vi "images.vi"(0 "Camera in":refnum<class "Camera.lvclass">, 1 "start_index":u32, 5 "data_format":T3(ring)=enum."Mono16", 7 "image_count":u32, 9 "crop":cluster{"x0":u64, "y0":u64, "x1":u64, "y1":u64}={"x0"=1, "y0"=1, "x1"=18446744073709551615, "y1"=18446744073709551615}, 11 "error in (no error)":errorcluster, 12 "PCO_Recorder_CompressionParams":T5={"dGainK"=nan, "dDarkNoise_e"=nan, "dDSNU_e"=nan, "dPRNU_pct"=nan, "dLightSourceNoise_pct"=0.0}) -> (2 "timestamp_list":T4(array[cluster]) {"lvTimestamp" format="%<%.6X\n%x>T"}, 3 "meta_data_list":T1(array[cluster]), 4 "Camera out":refnum<class "Camera.lvclass">, 6 "image_list (U8)":u8[][][](array[numeric]), 8 "image_list (U32)":u32[][][](array[numeric]), 10 "image_list (U64)":T2(array[cluster]), 13 "raw_image_8_list (U8)":u8[][][](array[numeric]), 14 "raw_image_list (U16)":u16[][][](array[numeric]), 15 "error out":errorcluster)   [LabVIEW 2019, in "Camera.lvclass"]
doc: "Get a series of images from the recorder as a 3D array. The positions of the images to query are defined by start_index and image_count. \nThis array is shaped depending on the\nresolution and ROI of the image and the number of recorded images. The data is stored in the\norder of image, row, column. The data format determines which output is valid, but the raw_image(16) output is always valid."
uses:
  Camera.lvclass
  Camera.lvclass/Camera.ctl
  pco.recorder/Recorder.lvlib
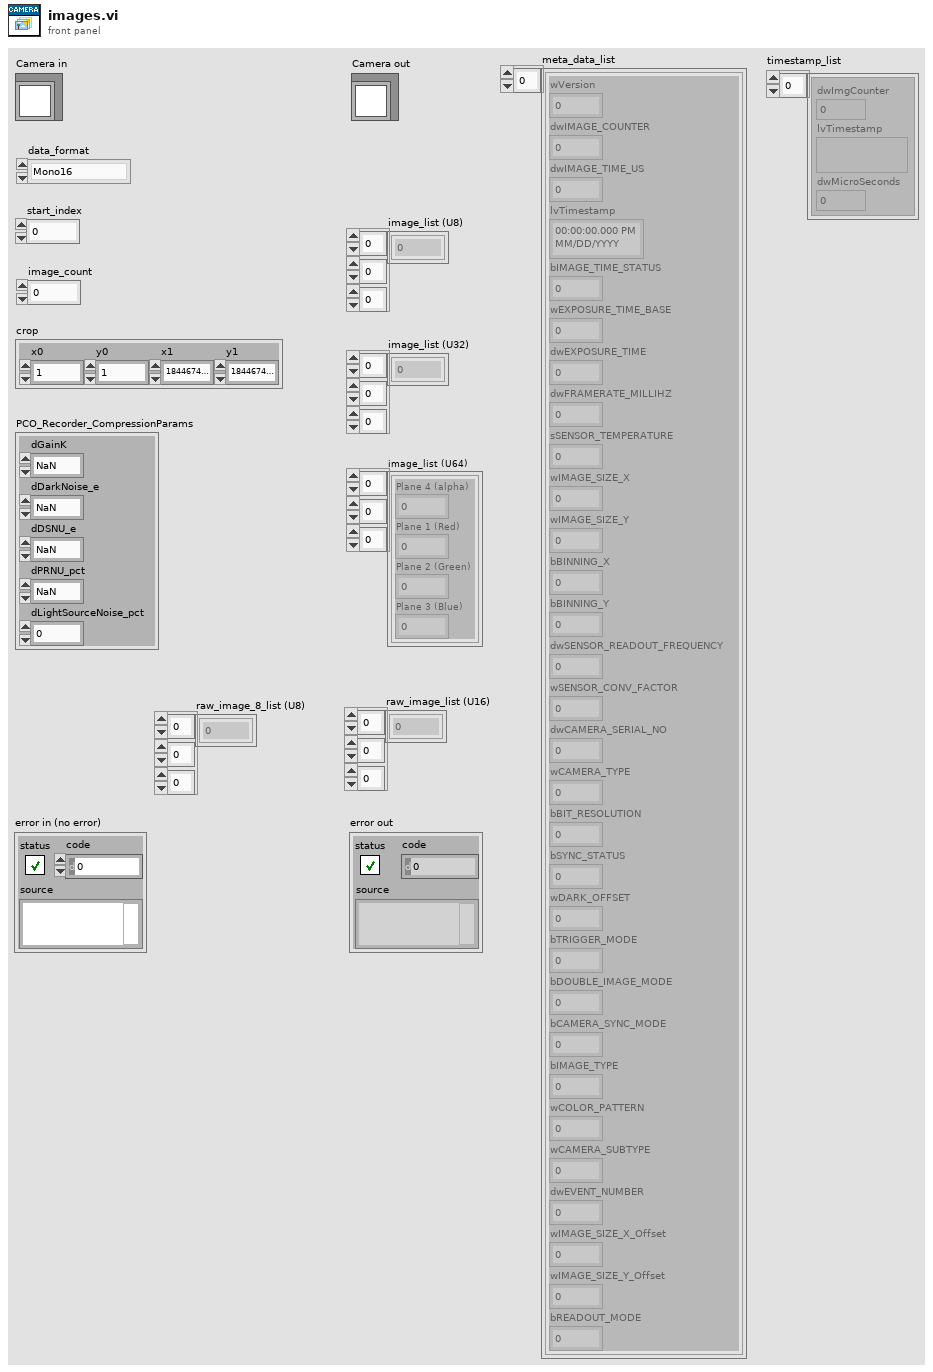
[diagram p1: front panel]
types:
  T1 = cluster{"wVersion":u16, "dwIMAGE_COUNTER":u32, "dwIMAGE_TIME_US":u32, "lvTimestamp":timestamp, "bIMAGE_TIME_STATUS":u8, "wEXPOSURE_TIME_BASE":u16, "dwEXPOSURE_TIME":u32, "dwFRAMERATE_MILLIHZ":u32, "sSENSOR_TEMPERATURE":i16, "wIMAGE_SIZE_X":u16, "wIMAGE_SIZE_Y":u16, "bBINNING_X":u8, "bBINNING_Y":u8, "dwSENSOR_READOUT_FREQUENCY":u32, "wSENSOR_CONV_FACTOR":u16, "dwCAMERA_SERIAL_NO":u32, "wCAMERA_TYPE":u16, "bBIT_RESOLUTION":u8, "bSYNC_STATUS":u8, "wDARK_OFFSET":u16, "bTRIGGER_MODE":u8, "bDOUBLE_IMAGE_MODE":u8, "bCAMERA_SYNC_MODE":u8, "bIMAGE_TYPE":u8, "wCOLOR_PATTERN":u16, "wCAMERA_SUBTYPE":u16, "dwEVENT_NUMBER":u32, "wIMAGE_SIZE_X_Offset":u16, "wIMAGE_SIZE_Y_Offset":u16, "bREADOUT_MODE":u8}[]
  T2 = cluster{"Plane 4 (alpha)":u16, "Plane 1 (Red)":u16, "Plane 2 (Green)":u16, "Plane 3 (Blue)":u16}[][][]
  T3 = enum16{"Undefined", "Mono8", "Mono16", "BGRA8", "RGBA8", "BGRA16", "RGBA16", "CompressedMono8"}
  T4 = cluster{"dwImgCounter":u32, "lvTimestamp":timestamp, "dwMicroSeconds":u32}[]
  T5 = cluster{"dGainK":dbl, "dDarkNoise_e":dbl, "dDSNU_e":dbl, "dPRNU_pct":dbl, "dLightSourceNoise_pct":dbl}
  T6 = cluster{"dwImgCounter":u32, "lvTimestamp":timestamp, "dwMicroSeconds":u32}
  T7 = cluster{"wVersion":u16, "dwIMAGE_COUNTER":u32, "dwIMAGE_TIME_US":u32, "lvTimestamp":timestamp, "bIMAGE_TIME_STATUS":u8, "wEXPOSURE_TIME_BASE":u16, "dwEXPOSURE_TIME":u32, "dwFRAMERATE_MILLIHZ":u32, "sSENSOR_TEMPERATURE":i16, "wIMAGE_SIZE_X":u16, "wIMAGE_SIZE_Y":u16, "bBINNING_X":u8, "bBINNING_Y":u8, "dwSENSOR_READOUT_FREQUENCY":u32, "wSENSOR_CONV_FACTOR":u16, "dwCAMERA_SERIAL_NO":u32, "wCAMERA_TYPE":u16, "bBIT_RESOLUTION":u8, "bSYNC_STATUS":u8, "wDARK_OFFSET":u16, "bTRIGGER_MODE":u8, "bDOUBLE_IMAGE_MODE":u8, "bCAMERA_SYNC_MODE":u8, "bIMAGE_TYPE":u8, "wCOLOR_PATTERN":u16, "wCAMERA_SUBTYPE":u16, "dwEVENT_NUMBER":u32, "wIMAGE_SIZE_X_Offset":u16, "wIMAGE_SIZE_Y_Offset":u16, "bREADOUT_MODE":u8}
  T8 = cluster{"Plane 4 (alpha)":u16, "Plane 1 (Red)":u16, "Plane 2 (Green)":u16, "Plane 3 (Blue)":u16}[][]
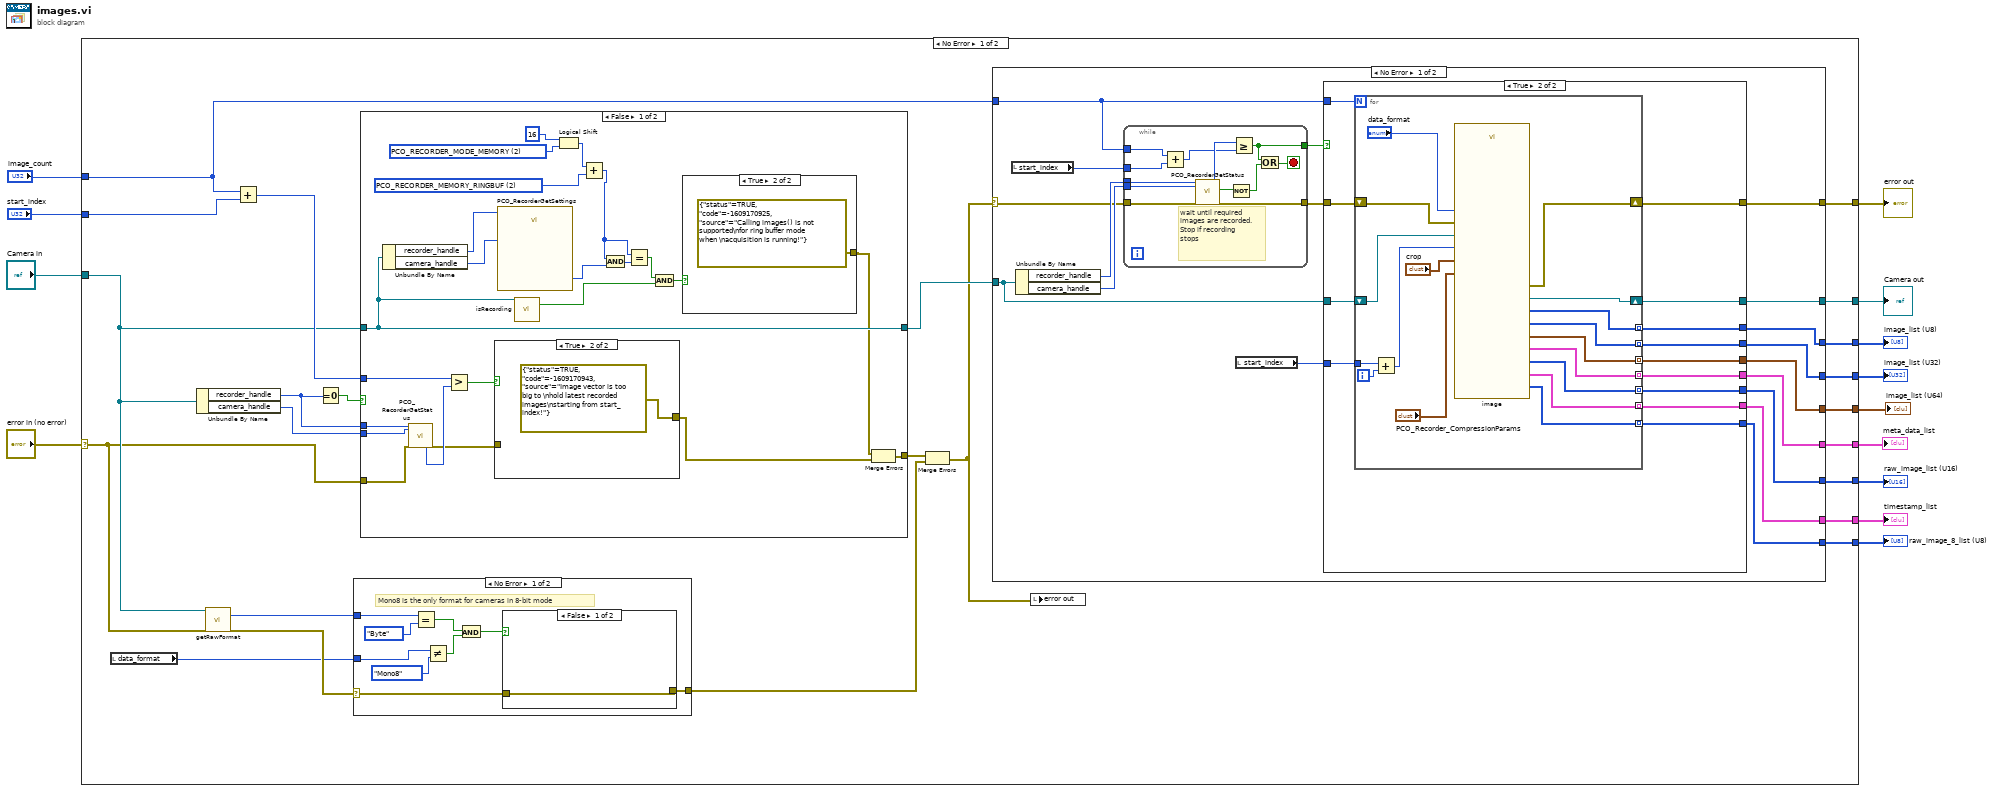
[diagram p0: block diagram]
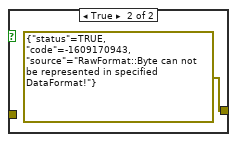
[diagram p2: hidden frame]
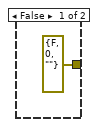
[diagram p4: hidden frame]
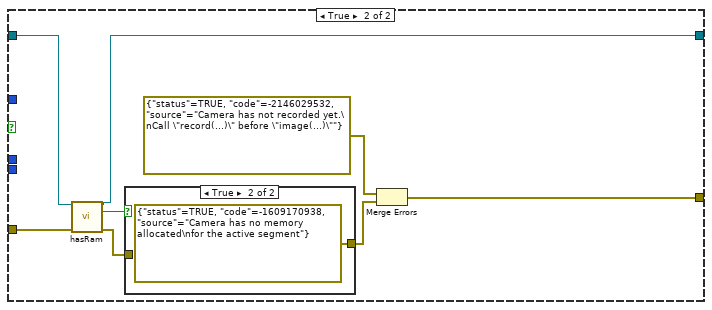
[diagram p6: hidden frame]
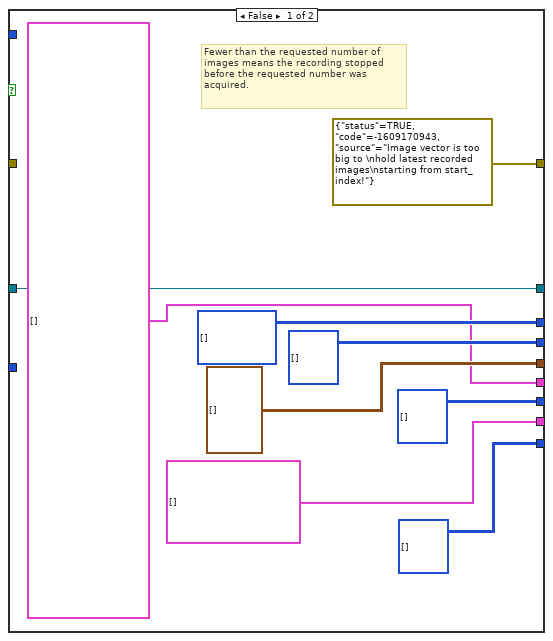
[diagram p8: hidden frame]
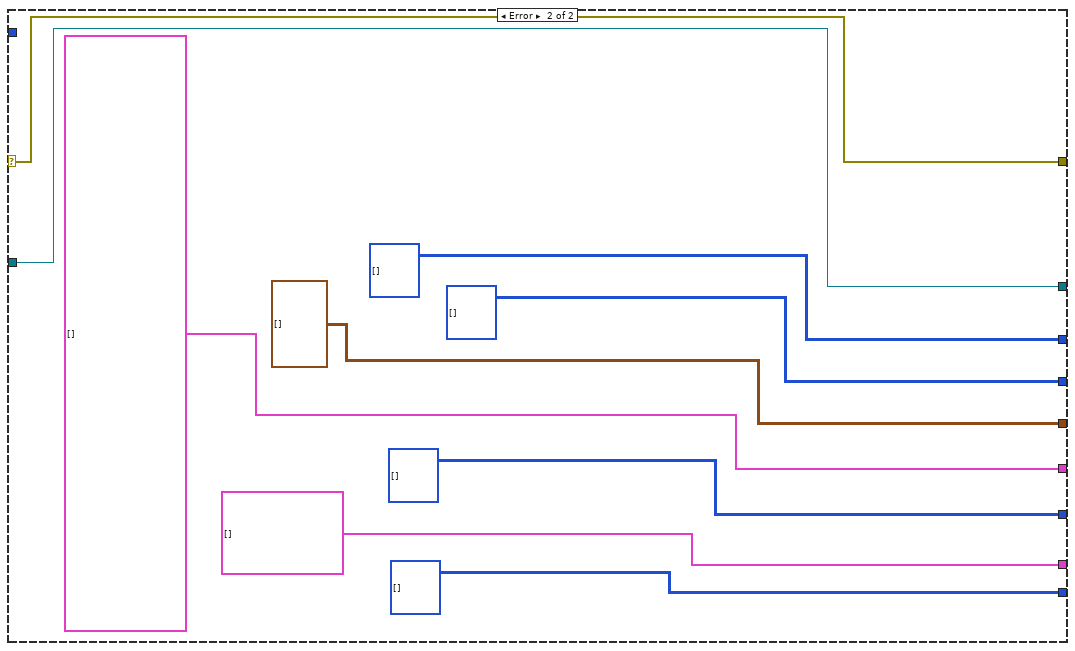
[diagram p9: hidden frame]
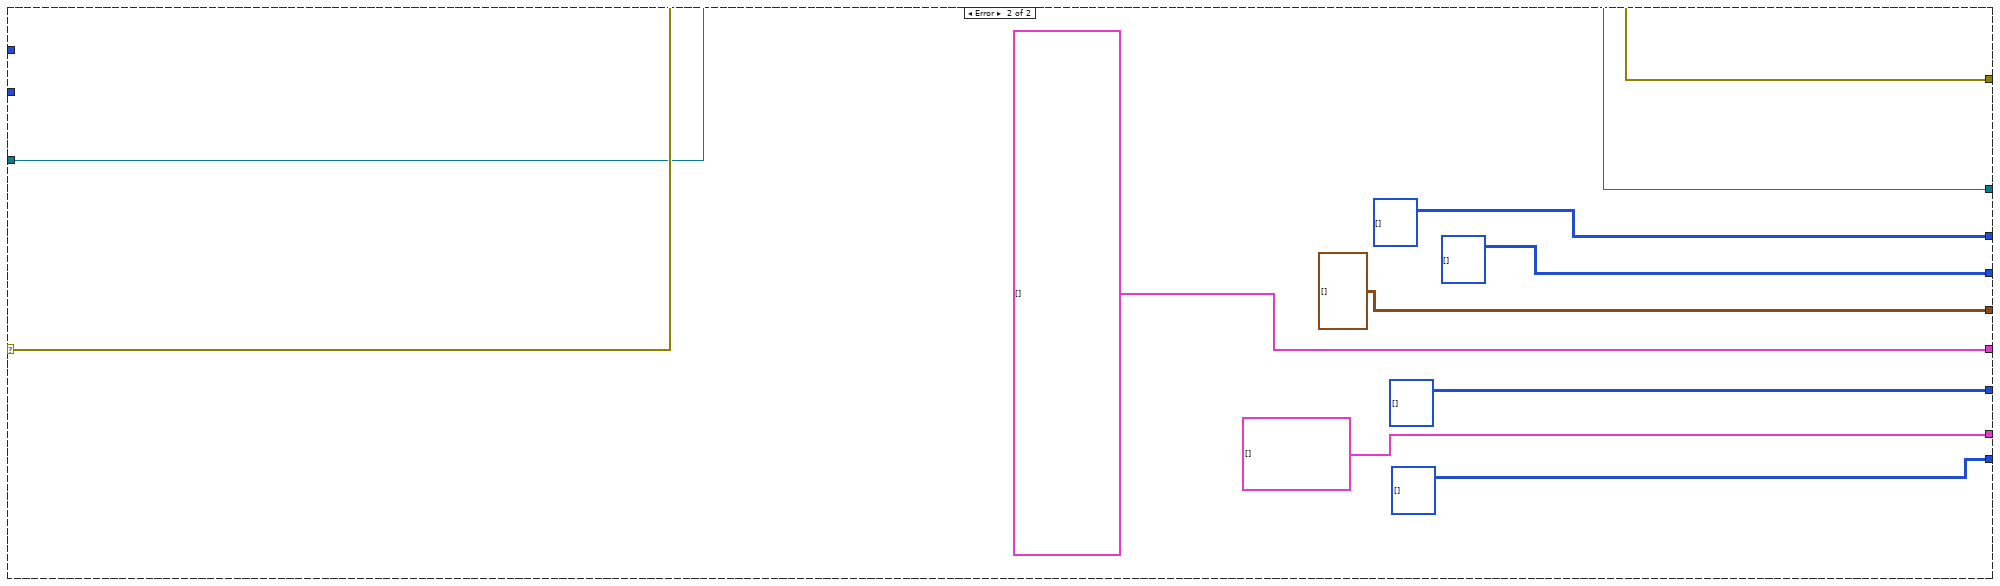
[diagram p10: hidden frame]
diagram:
  n1 = case shown="No Error" "error in (no error)" {
    selector: "error in (no error)" -> [w15 w171]
    tunnel: "Camera in" -> [w16 w170]
    tunnel: "image_count" -> [w29 _]
    tunnel: [w37 w171] -> w10
    tunnel: [w36 w170] -> w9
    tunnel: [w35 u8[][][] [] ("image (U8)")] -> w8
    tunnel: [w34 u32[][][] [] ("image (U16)")] -> w7
    tunnel: [w33 T1 [] ("meta_data_list")] -> w1
    tunnel: [w32 u16[][][] [] ("raw_image (U16)")] -> w6
    tunnel: [w31 T4 []] -> w5
    tunnel: "start_index" -> [w30 _]
    tunnel: [w28 T2 [] ("image (U64)")] -> w3
    tunnel: [w14 u8[][][] [] ("raw_image (U16)")] -> w2
    frame No Error {
      n2 = local read "data_format"() -> (w19:T3)
      n3 = Unbundle By Name(w16) -> ("recorder_handle"=w26:u64, "camera_handle"=w25:u64)
      n4 = call-dynamic "getRawFormat.vi"("Camera in"=w16, "error in (no error)"=w15) -> ("rawFormat"=w20:enum16{"Word", "Byte"}, "error out"=w21:errorcluster)  [unwired: 11 in, 1 out]
      n5 = Add(x=w29, y=w30) -> (x+y=w24:u32)
      n6 = Equal To 0?(x=w26) -> (x = 0?=w27:bool)
      n7 = case shown="No Error" w21 {
        selector: w21 -> [w39 w49]
        tunnel: w20 -> [w46 _]
        tunnel: w19 -> [w44 _]
        tunnel: [w38 w49] -> w17
        frame No Error {
          # "Mono8 is the only format for cameras in 8-bit mode"
          n8 = Equal?(x=w46, y=enum16{"Word", "Byte"}."Byte" ("rawFormat")) -> (x = y?=w42:bool)
          n9 = Not Equal?(x=w44, y=T3."Mono8" ("data_format")) -> (x != y?=w41:bool)
          n10 = And(x=w42, y=w41) -> (x .and. y?=w40:bool)
          n11 = case shown="False" w40 {
            tunnel: w39 -> [w47 _]
            tunnel: [w47 errorcluster {"status"=TRUE, "code"=-1609170943, "source"="RawFormat::Byte can not be represented in specified DataFormat!"} ("error constant")] -> w38
            frame False {
            }
            frame True {
            }
          }
        }
        frame Error {
        }
      }
      n12 = case shown="False" w27 {
        tunnel: w15 -> [w72 w80]
        tunnel: w16 -> [w59 w79]
        tunnel: [w57 w78] -> w22
        tunnel: w26 -> [w71 _]
        tunnel: w25 -> [w70 _]
        tunnel: w24 -> [w69 _]
        tunnel: [w59 w77] -> w23
        frame False {
          w50 = u32 2 items=["PCO_RECORDER_MODE_FILE"=1, "PCO_RECORDER_MODE_MEMORY"=2, "PCO_RECORDER_MODE_CAMRAM"=3] ("wRecMode")
          w62 = u32 2 items=["PCO_RECORDER_MEMORY_SEQUENCE"=1, "PCO_RECORDER_MEMORY_RINGBUF"=2, "PCO_RECORDER_MEMORY_FIFO"=3] ("wRecType")
          n13 = Unbundle By Name(w59) -> ("recorder_handle"=w65:u64, "camera_handle"=w64:u64)
          n14 = call "PCO_RecorderGetStatus.vi"("phRec"=w71, "phCam"=w70, "error in (no error)"=w72) -> ("dwReqImgCount"=w68:u32, "error out"=w66:errorcluster)  [unwired: 5 in, 10 out]
          n15 = Greater?(x=w69, y=w68) -> (0:w67:bool)
          n16 = case shown="True" w67 {
            tunnel: [w75 errorcluster {"status"=TRUE, "code"=-1609170943, "source"="Image vector is too big to \nhold latest recorded images\nstarting from start_index!"} ("error constant")] -> w56
            tunnel: w66 -> [w75 _]
            frame False {
            }
            frame True {
            }
          }
          n17 = call "PCO_RecorderGetSettings.vi"("phRec"=w65, "phCam"=w64) -> ("dwRecMode"=w54:u32)  [unwired: 5 in, 8 out]
          n18 = call-dynamic "isRecording.vi"("Camera in"=w59) -> ("recording"=w60:bool)  [unwired: 12 in, 2 out]
          n19 = Logical Shift(y=u32 16 ("x"), x=w50) -> (x << y=w63:u32)
          n20 = Add(x=w63, y=w62) -> (x+y=w52:u32)
          n21 = And(x=w52, y=w54) -> (x .and. y?=w53:u32)
          n22 = Equal?(x=w52, y=w53) -> (x = y?=w61:bool)
          n23 = And(x=w61, y=w60) -> (x .and. y?=w58:bool)
          n24 = case shown="True" w58 {
            tunnel: [errorcluster {"status"=FALSE, "code"=0, "source"=""} ("error constant") errorcluster {"status"=TRUE, "code"=-1609170925, "source"="Calling images() is not supported\nfor ring buffer mode when \nacquisition is running!"} ("error constant")] -> w55
            frame False {
            }
            frame True {
            }
          }
          n25 = Merge Errors(w55, w56) -> (w57:errorcluster)
        }
        frame True {
          n26 = call-dynamic "hasRam.vi"("Camera in"=w79, "error in (no error)"=w80) -> ("Camera out"=w77:refnum<class "Camera.lvclass">, "hasRam"=w84:bool, "error out"=w83:errorcluster)  [unwired: 11 in]
          n27 = case shown="True" w84 {
            tunnel: w83 -> [w85 _]
            tunnel: [w85 errorcluster {"status"=TRUE, "code"=-1609170938, "source"="Camera has no memory allocated\nfor the active segment"} ("error constant")] -> w81
            frame False {
            }
            frame True {
            }
          }
          n28 = Merge Errors(errorcluster {"status"=TRUE, "code"=-2146029532, "source"="Camera has not recorded yet.\nCall \"record(...)\" before \"image(...)\""} ("error constant"), w81) -> (w78:errorcluster)
        }
      }
      n29 = Merge Errors(w22, w17) -> (w18:errorcluster)
      n30 = case shown="No Error" w18 {
        selector: w18 -> [w92 w164]
        tunnel: w29 -> [w102 _]
        tunnel: w23 -> [w101 w163]
        tunnel: [w99 w164] -> w37
        tunnel: [w98 w163] -> w36
        tunnel: [w93 u8[][][] [] ("image (U8)")] -> w35
        tunnel: [w97 u32[][][] [] ("image (U16)")] -> w34
        tunnel: [w89 T2 [] ("image (U64)")] -> w28
        tunnel: [w96 T1 [] ("meta_data_list")] -> w33
        tunnel: [w95 u16[][][] [] ("raw_image (U16)")] -> w32
        tunnel: [w94 T4 []] -> w31
        tunnel: [w87 u8[][][] [] ("raw_image (U16)")] -> w14
        frame No Error {
          n31 = local read "start_index"() -> (w91:u32)
          n32 = Unbundle By Name(w101) -> ("recorder_handle"=w104:u64, "camera_handle"=w103:u64)
          n33 = while {
            tunnel: w104 -> [w155]
            tunnel: w103 -> [w154]
            tunnel: w92 -> [w153]
            tunnel: w102 -> [w150]
            tunnel: [w152] -> w100
            tunnel: w91 -> [w149]
            tunnel: [w144] -> w88
            stop <- w145 stop-if-true
            # "wait until required \nimages are recorded. Stop if recording stops"
            n34 = Add(x=w150, y=w149) -> (x+y=w148:u32)
            n35 = call "PCO_RecorderGetStatus.vi"("phRec"=w155, "phCam"=w154, "error in (no error)"=w153) -> ("dwProcImgCount"=w151:u32, "bIsRunning"=w147:bool, "error out"=w152:errorcluster)  [unwired: 5 in, 9 out]
            n36 = Not(x=w147) -> (.not. x?=w146:bool)
            n37 = Greater Or Equal?(x=w151, y=w148) -> (x >= y?=w144:bool)
            n38 = Or(x=w144, y=w146) -> (x .or. y?=w145:bool)
          }
          n39 = local read "start_index"() -> (w90:u32)
          n40 = case shown="True" w88 {
            tunnel: w102 -> [_ w126]
            tunnel: w101 -> [w112 w125]
            tunnel: w100 -> [_ w124]
            tunnel: [errorcluster {"status"=TRUE, "code"=-1609170943, "source"="Image vector is too big to \nhold latest recorded images\nstarting from start_index!"} ("error constant") w123] -> w99
            tunnel: [w112 w122] -> w98
            tunnel: [u32[][][] [] ("image (U32)") w121] -> w97
            tunnel: [T1 [] ("meta_data_list") w120] -> w96
            tunnel: [u16[][][] [] ("raw_image (U16)") w119] -> w95
            tunnel: [T4 [] w118] -> w94
            tunnel: [u8[][][] [] ("image (U8)") w117] -> w93
            tunnel: w90 -> [_ w116]
            tunnel: [T2 [] ("image (U64)") w115] -> w89
            tunnel: [u8[][][] [] ("raw_image (U16)") w114] -> w87
            frame False {
              # "Fewer than the requested number of images means the recording stopped before the requested number was acquired."
            }
            frame True {
              n41 = for {
                N: w126 -> [_]
                shift-right: [w140] -> w123
                shift-left: w124 -> [w141]
                shift-right: [w139] -> w122
                shift-left: w125 -> [w143]
                tunnel: [w138] -> w121 mode=indexing
                tunnel: [w137] -> w117 mode=indexing
                tunnel: [w136] -> w115 mode=indexing
                tunnel: [w135] -> w120 mode=indexing
                tunnel: [w134] -> w119 mode=indexing
                tunnel: [w131] -> w118 mode=indexing
                tunnel: w116 -> [w129]
                tunnel: [w127] -> w114 mode=indexing
                i -> [w130]
                n42 = Add(x=w129, y=w130) -> (x+y=w128:u32)
                n43 = call-dynamic "image.vi"("Camera in"=w143, "data_format"="data_format", "image_index"=w128, "crop"="crop", "error in (no error)"=w141, "PCO_Recorder_CompressionParams"="PCO_Recorder_CompressionParams") -> ("timestamp"=w131:T6, "meta_data"=w135:T7, "Camera out"=w139:refnum<class "Camera.lvclass">, "image (U8)"=w137:u8[][], "image (U32)"=w138:u32[][], "image (U64)"=w136:T8, "raw_image_8bit (U8)"=w127:u8[][], "raw_image (U16)"=w134:u16[][], "error out"=w140:errorcluster)  [unwired: 1 in]
              }
            }
          }
        }
        frame Error {
        }
      }
      n44 = local write "error out"(w18) -> ()
    }
    frame Error {
    }
  }
  "error out" <- w10
  "Camera out" <- w9
  "timestamp_list" <- w5
  "raw_image_list (U16)" <- w6
  "image_list (U32)" <- w7
  "image_list (U8)" <- w8
  "image_list (U64)" <- w3
  "raw_image_8_list (U8)" <- w2
  "meta_data_list" <- w1
